vi "LWXPS_EventExtendedConfigurationTriggerSet.vi"(0 "Extended Event Name IN":string[](array[string]), 1 "Event Parameter 1 IN":string[](array[string]), 2 "Event Parameter 2 IN":string[](array[string]), 3 "Event Parameter 3 IN":string[](array[string]), 4 "Event Parameter 4 IN":string[](array[string]), 5 "LabVIEW error IN":errorcluster, 6 "XPS Reference IN":refnum<k24>) -> (10 "XPS Reference OUT":refnum<k24>, 12 "Returned error code":i32, 13 "LabVIEW error OUT":errorcluster, 14 "Extended Event Name OUT":string[](array[string]), 15 "Event Parameter 1 OUT":string[](array[string]), 16 "Event Parameter 2 OUT":string[](array[string]), 17 "Event Parameter 3 OUT":string[](array[string]), 18 "Event Parameter 4 OUT":string[](array[string]), 19 "XPS Error String":string)   [LabVIEW 2014]
uses:
  D:/XPSQ8_LabView_Library/Development/Source/Dll/Newport.XPS.CommandInterface.dll
  Dll/Newport.XPS.CommandInterface.dll
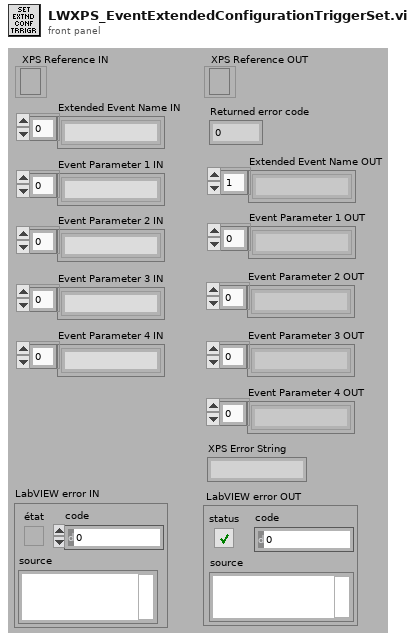
[diagram p1: front panel]
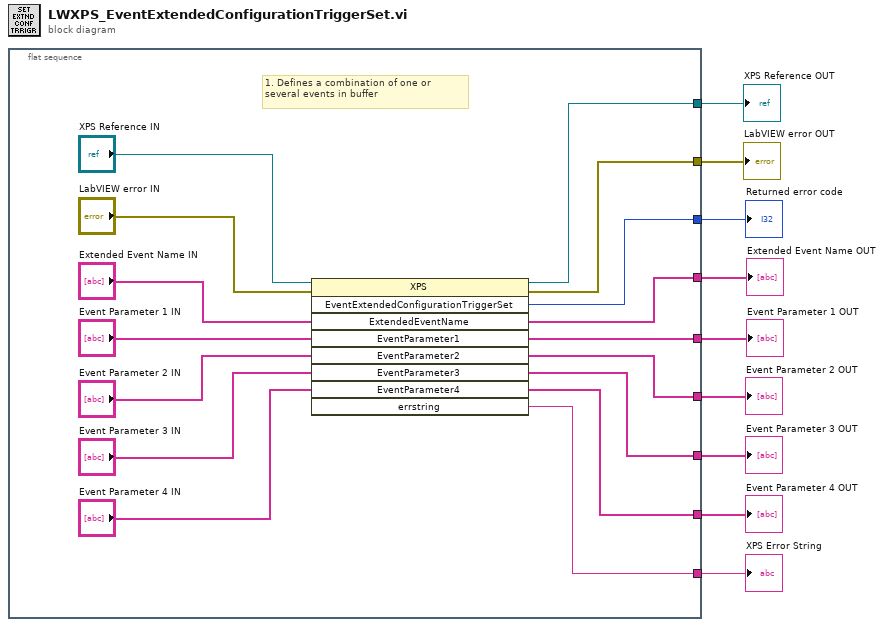
[diagram p0: block diagram]
diagram:
  n1 = flat-sequence {
    tunnel: [w23] -> w9
    tunnel: [w22] -> w8
    tunnel: [w21] -> w7
    tunnel: [w20] -> w1
    tunnel: [w19] -> w6
    tunnel: [w18] -> w5
    tunnel: [w17] -> w4
    tunnel: [w16] -> w3
    tunnel: [w11] -> w2
    frame #0 {
      # "1. Defines a combination of one or several events in buffer"
      n2 = invoke class="XPS" method="EventExtendedConfigurationTriggerSet"(reference="XPS Reference IN", error in="LabVIEW error IN", "ExtendedEventName"="Extended Event Name IN", "EventParameter1"="Event Parameter 1 IN", "EventParameter2"="Event Parameter 2 IN", "EventParameter3"="Event Parameter 3 IN", "EventParameter4"="Event Parameter 4 IN") -> (reference out=w23:refnum<k24>, error out=w22:errorcluster, "EventExtendedConfigurationTriggerSet"=w21:i32, "ExtendedEventName"=w11:string[], "EventParameter1"=w20:string[], "EventParameter2"=w19:string[], "EventParameter3"=w18:string[], "EventParameter4"=w17:string[], "errstring"=w16:string)  [unwired: 2 in]
    }
  }
  "XPS Reference OUT" <- w9
  "LabVIEW error OUT" <- w8
  "Returned error code" <- w7
  "Event Parameter 2 OUT" <- w6
  "Event Parameter 3 OUT" <- w5
  "Event Parameter 4 OUT" <- w4
  "XPS Error String" <- w3
  "Extended Event Name OUT" <- w2
  "Event Parameter 1 OUT" <- w1
